vi "Wait Logic.vi"(8 "error in (no error)":errorcluster, 11 "Time":string) -> (0 "error out":errorcluster, 1 "Status String":string, 2 "timer value":u32, 3 "Trigger":bool)   [LabVIEW 2019, in "Instrument.lvlib" / "Instrument.lvclass"]
doc: "Use to control a non-blocking Wait sequence.\n\n<B>Time</B>: Time to wait in milliseconds.\nIf <B>Time</B> = <B>\"\"</B> or <B>RESET</B> the counter will reset and the Trigger output will be TRUE."
uses:
  Instrument.lvclass
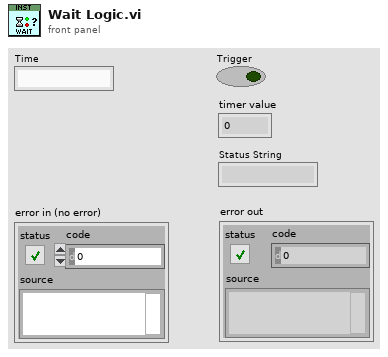
[diagram p1: front panel]
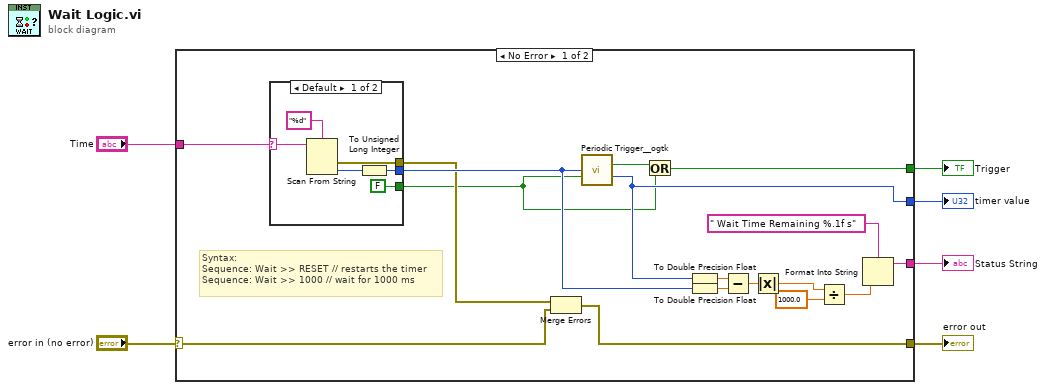
[diagram p0: block diagram]
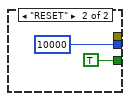
[diagram p2: hidden frame]
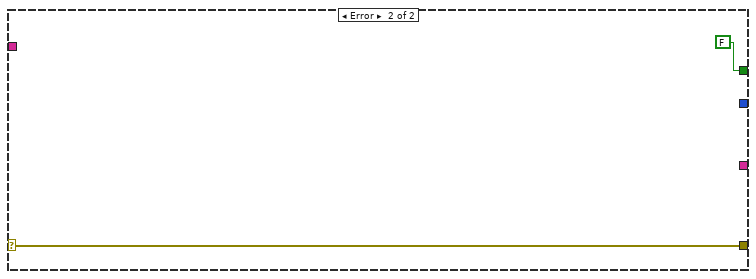
[diagram p3: hidden frame]
diagram:
  n1 = case shown="No Error" "error in (no error)" {
    selector: "error in (no error)" -> [w10 w33]
    tunnel: [w19 _] -> w6
    tunnel: [w18 FALSE] -> w5
    tunnel: [w9 w33] -> w3
    tunnel: "Time" -> [w13 _]
    tunnel: [w8 _] -> w1
    frame No Error {
      # "Syntax:\nSequence: Wait >> RESET // restarts the timer\nSequence: Wait >> 1000 // wait for 1000 ms"
      n2 = case shown="Default" w13 {
        selector: w13 -> [w26 _]
        tunnel: [w28 u32 10000 ("time (ms)")] -> w12
        tunnel: [FALSE ("reset") TRUE ("reset")] -> w7
        tunnel: [w24 _] -> w11
        frame Default {
          n3 = Scan From String(format string="%d", input string=w26) -> (error out=w24:errorcluster, output 1=w27:i32)  [unwired: 3 in, 2 out]
          n4 = To Unsigned Long Integer(number=w27) -> (unsigned 32bit integer=w28:u32)
        }
        frame "RESET" {
        }
      }
      n5 = Merge Errors(w11, w10) -> (w9:errorcluster)
      n6 = call <userlib>:"Periodic Trigger__ogtk.vi"("time (ms)"=w12, "reset"=w7) -> ("Triggered"=w14:bool, "timer value"=w8:u32)  [unwired: 11 in, 1 out]
      n7 = Or(x=w14, y=w7) -> (x .or. y?=w18:bool)
      n8 = To Double Precision Float(number=w8) -> (double precision float=w22:dbl)
      n9 = To Double Precision Float(number=w12) -> (double precision float=w23:dbl)
      n10 = Subtract(x=w22, y=w23) -> (x-y=w21:dbl)
      n11 = Absolute Value(x=w21) -> (abs(x)=w20:dbl)
      n12 = Divide(x=w20, y=1000.0) -> (x/y=w16:dbl)
      n13 = Format Into String(format string=" Wait Time Remaining %.1f s", w16) -> (resulting string=w19:string)  [unwired: 2 in, 1 out]
    }
    frame Error {
    }
  }
  "Status String" <- w6
  "Trigger" <- w5
  "error out" <- w3
  "timer value" <- w1
